vi "FindLineAndOverwrite.vi"(0 "Exposure path":path, 5 "Name":string, 7 "Index":u32, 9 "Exposure":u32, 11 "error in (no error)":errorcluster) -> (15 "error out":errorcluster)   [LabVIEW 2013]
panel:
  out "match substring":string
  out "Input String":string
  out "Output string":string
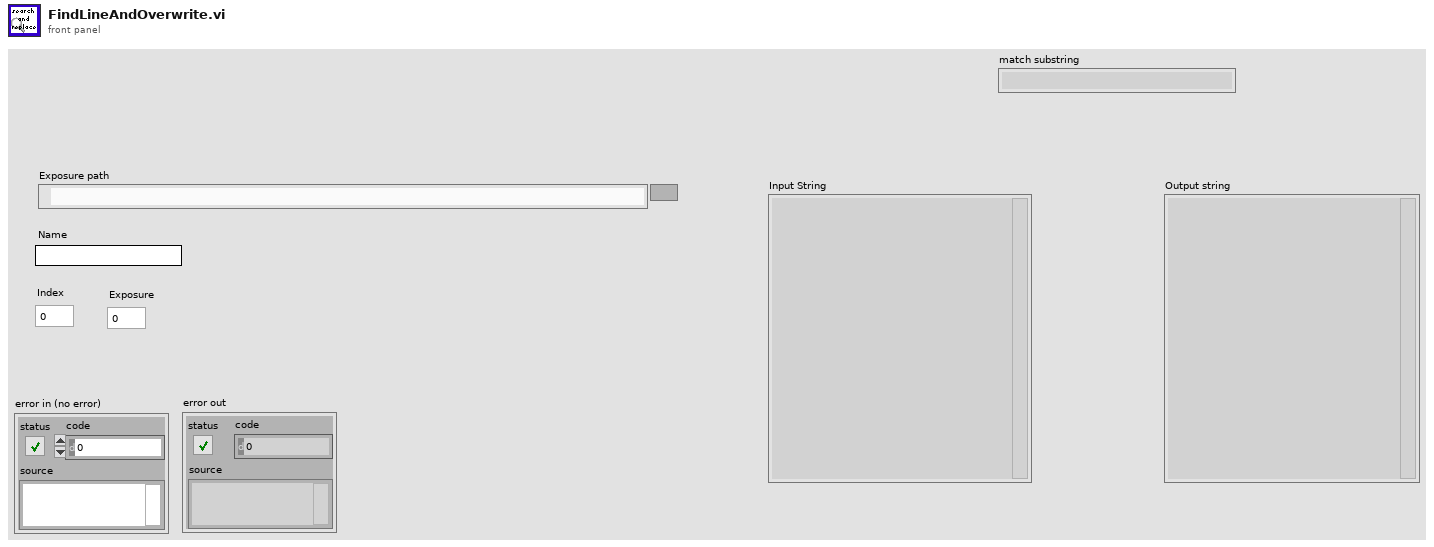
[diagram p1: front panel]
types:
  T1 = enum16{"open", "replace", "create", "open or create", "replace or create", "replace or create with confirmation"}
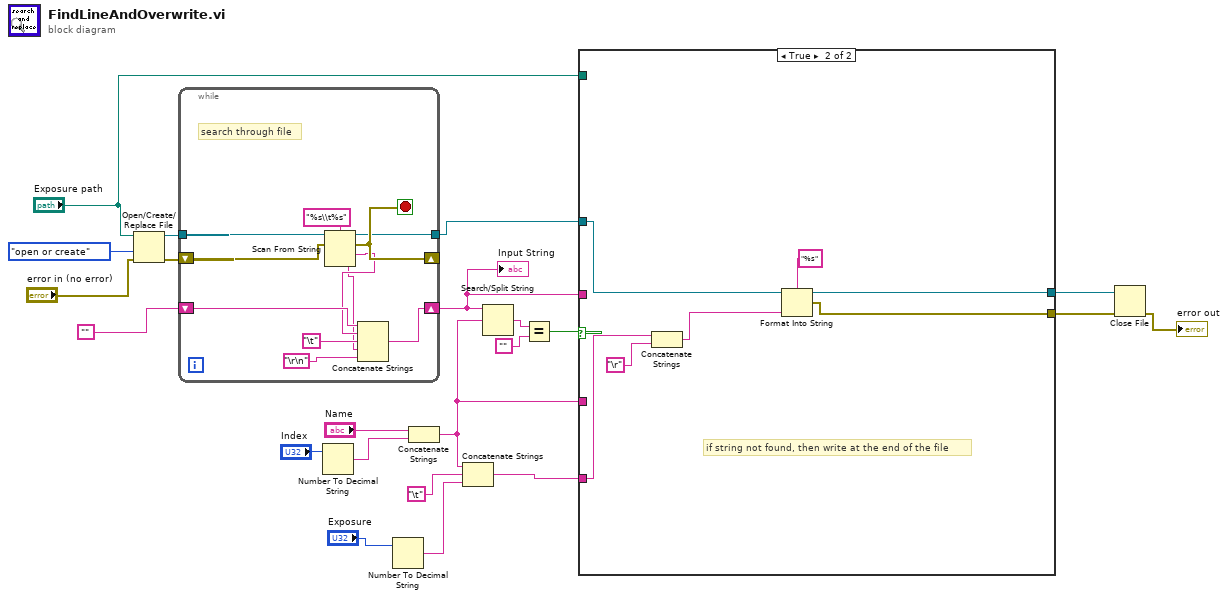
[diagram p0: block diagram]
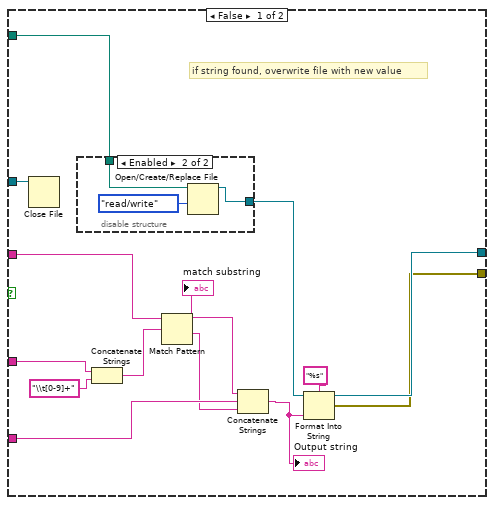
[diagram p2: hidden frame]
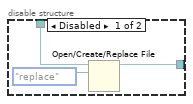
[diagram p3: hidden frame]
diagram:
  n1 = Open/Create/Replace File(file path (use dialog)="Exposure path", error in="error in (no error)", operation (0:open)=T1."open or create") -> (refnum out=w16:refnum<file>, error out=w15:errorcluster)  [unwired: 3 in, 1 out]
  n2 = while {
    tunnel: w16 -> [w32]
    shift-right: [w30] -> _
    shift-left: w15 -> [w31]
    shift-right: [w29] -> w5
    shift-left: "" -> [w27]
    tunnel: [w28] -> w9
    stop <- w30 stop-if-true
    # "search through file"
    n3 = Scan From String("%s\\t%s" ("format string"), w32, w31) -> (w28:refnum<file>, w30:errorcluster, output 1=w26:string, output 2=w24:string)  [unwired: 2 in]
    n4 = Concatenate Strings(w27, w26, "\t", w24, "\r\n") -> (w29:string)
  }
  "Input String" <- w5
  n5 = Number To Decimal String(number="Index") -> (decimal integer string=w21:string)  [unwired: 1 in]
  n6 = Number To Decimal String(number="Exposure") -> (decimal integer string=w7:string)  [unwired: 1 in]
  n7 = Concatenate Strings("Name", w21) -> (w2:string)
  n8 = Concatenate Strings(w2, "\t", w7) -> (w6:string)
  n9 = Search/Split String(string=w5, search string/char (-)=w2) -> (match + rest of string=w12:string)  [unwired: 1 in, 2 out]
  n10 = Equal?(x=w12, y="") -> (x = y?=w10:bool)
  n11 = case shown="True" w10 {
    tunnel: w9 -> [w48 w60]
    tunnel: w6 -> [w43 w57]
    tunnel: w5 -> [w47 _]
    tunnel: [w39 w59] -> w4
    tunnel: [w38 w58] -> w3
    tunnel: w2 -> [w46 _]
    tunnel: "Exposure path" -> [w41 _]
    frame False {
      # "if string found, overwrite file with new value"
      n12 = Close File(refnum=w48) -> ()  [unwired: 1 in, 2 out]
      n13 = disable-structure shown="Enabled" {
        disable-tunnel: w41 -> [w50 w53]
        disable-tunnel: [w49 w52] -> w40
        frame Disabled {
          n14 = Open/Create/Replace File(file path (use dialog)=w50, operation (0:open)=T1."replace") -> (refnum out=w49:refnum<file>)  [unwired: 4 in, 2 out]
        }
        frame Enabled {
          n15 = Open/Create/Replace File(file path (use dialog)=w53, access (0:read/write)=enum16{"read/write", "read-only", "write-only"}."read/write") -> (refnum out=w52:refnum<file>)  [unwired: 4 in, 2 out]
        }
      }
      n16 = Concatenate Strings(w46, "\\t[0-9]+" ("regular expression")) -> (w45:string)
      n17 = Match Pattern(string=w47, regular expression=w45) -> (before substring=w44:string, match substring=→"match substring":string, after substring=w42:string)  [unwired: 1 in, 1 out]
      n18 = Concatenate Strings(w44, w43, w42) -> (w34:string)
      "Output string" <- w34
      n19 = Format Into String(format string="%s" ("format (%.3f)"), initial string=w40, w34) -> (resulting string=w39:refnum<file>, error out=w38:errorcluster)  [unwired: 1 in]
    }
    frame True {
      # "if string not found, then write at the end of the file"
      n20 = Concatenate Strings(w57, "\r") -> (w55:string)
      n21 = Format Into String(format string="%s" ("format (%.3f)"), initial string=w60, w55) -> (resulting string=w59:refnum<file>, error out=w58:errorcluster)  [unwired: 1 in]
    }
  }
  n22 = Close File(refnum=w4, error in=w3) -> (error out=→"error out":errorcluster)  [unwired: 1 out]
